vi "ABCD to S - 2nPort.vi"(8 "error in (no error)":errorcluster, 10 "Zc (Ohm)":cdb[](array[numeric]), 11 "ABCD Array In":cdb[][](array[numeric])) -> (0 "error out":errorcluster, 3 "S-par Array Out":cdb[][](array[numeric]))   [LabVIEW 2023, in "NI_HFNetworkAnalysis.lvlib"]
doc: "Convert a 2N-port ABCD array to an S-parameter array, where the characteristic impedance Zc is specified for each port:\n<b>{ b1, b2, b3, b4 } = S . { a1, a2, a3, a4 }</b>\n\nInput ABCD array rows are defined as <b>(a11,a12,a13,a14,...,a21,a22,a23,a24,...,a31,a32,a33,a34,...,a41,a42,a43,a44,...)</b>\nand output S-parameter array rows are defined as <b>(S11,S12,S13,S14,...,S21,S22,S23,S24,...,S31,S32,S33,S34,...,S41,S42,S43,S44,...)</b>.\n\n<b>Note</b>\nThe convention for both S-parameters and ABCD arrays for the current is <b>\"positive when flowing into the port\"</b>.\n\n<b>Known Limitations</b>\nTransformation supports only 2n-port networks."
uses:
  NI_HFNetworkAnalysis.lvlib
  <vilib>/Analysis/baseanly.llb/Complex A x B.vi
  <vilib>/Analysis/Matrix/Numeric/Conversions/Array To Matrix - CA2.vi
  <vilib>/Analysis/baseanly.llb/Complex Inverse Matrix.vi
  <vilib>/Analysis/Matrix/Numeric/Conversions/Matrix To Array - CM.vi
  <vilib>/Analysis/Matrix/NI_Matrix.lvlib
  <vilib>/Analysis/NI_AALBase.lvlib
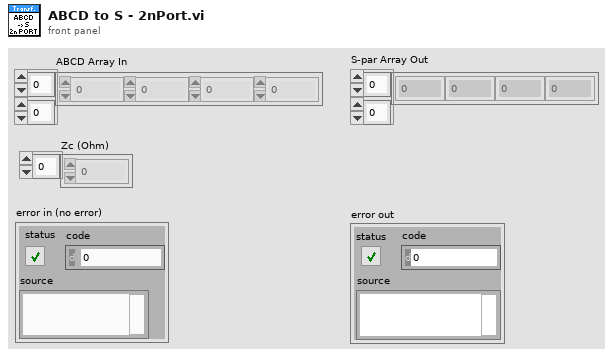
[diagram p1: front panel]
types:
  T1 = typedef "NI_Matrix.lvlib/ComplexMatrix.ctl" = cdb[][]
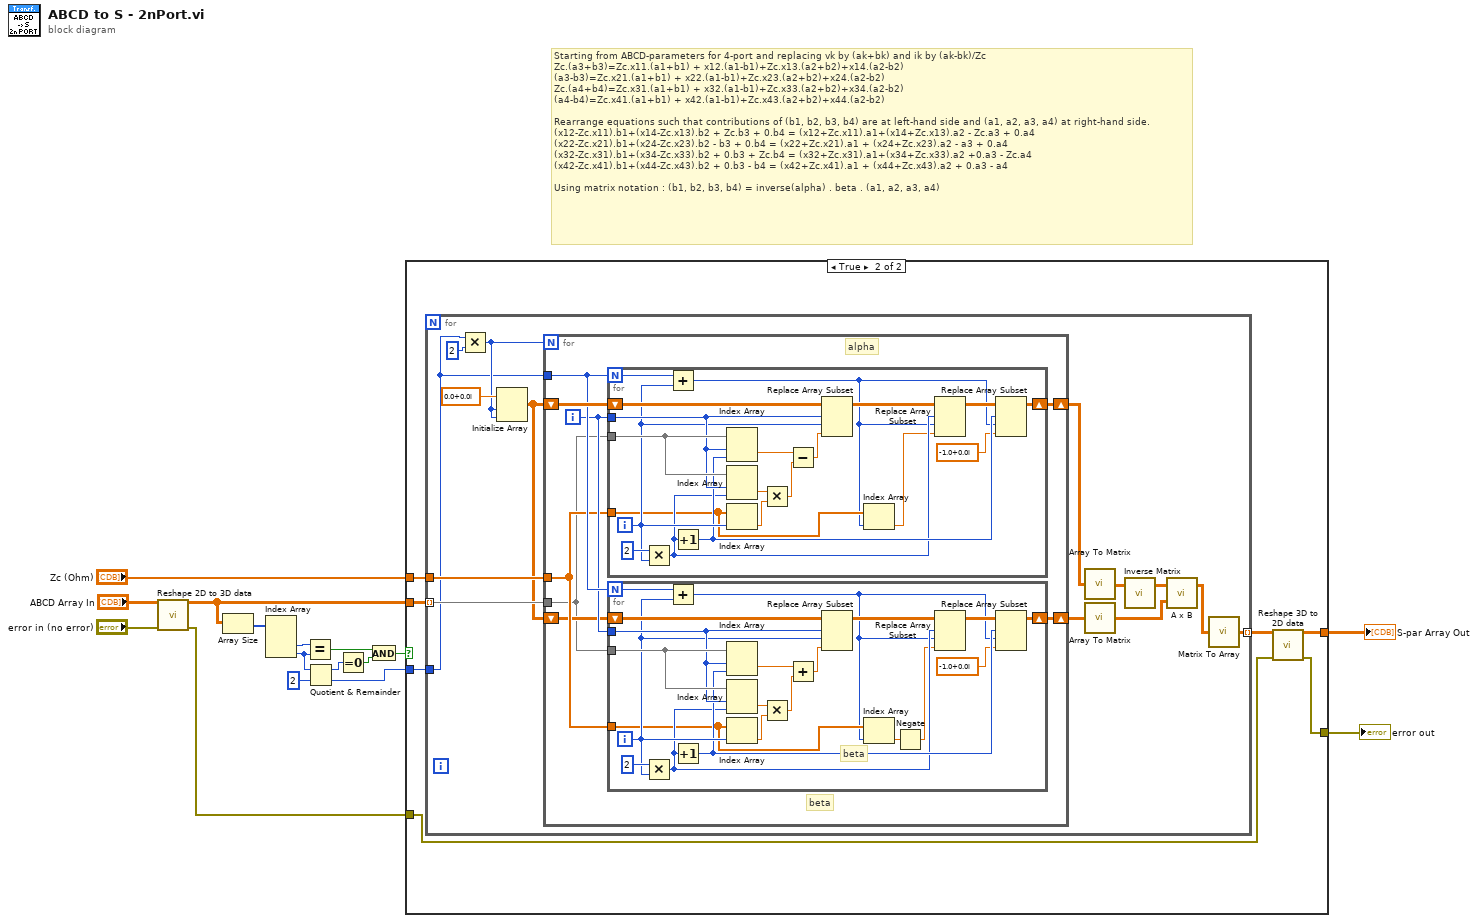
[diagram p0: block diagram]
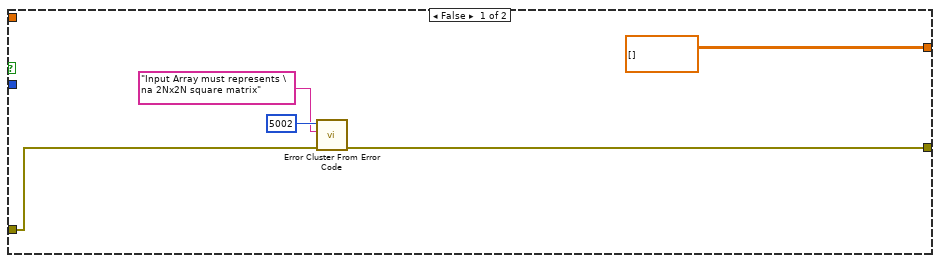
[diagram p2: hidden frame]
diagram:
  # "Starting from ABCD-parameters for 4-port and replacing vk by (ak+bk) and ik by (ak-bk)/Zc\nZc.(a3+b3)=Zc.x11.(a1+b1) + x12.(a1-b1)+Zc.x13.(a2+b2)+x14.(a2-b2)\n(a3-b3)=Zc.x21.(a1+b1) + x22.(a1-b1)+Zc.x23.(a2+b2)+x24.(a2-b2)\nZc.(a4+b4)=Zc.x31.(a1+b1) + x32.(a1-b1)+Zc.x33.(a2+b2)+x34.(a2-b2)\n(a4-b4)=Zc.x41.(a1+b1) + x42.(a1-b1)+Zc.x43.(a2+b2)+x44.(a2-b2)\n\nRearrange equations such that contributions of (b1, b2, b3, b4) are at left-hand side and (a1, a2, a3, a4) at right-hand side.\n(x12-Zc.x11).b1+(x14-Zc.x13).b2 + Zc.b3 + 0.b4 = (x12+Zc.x11).a1+(x14+Zc.x13).a2 - Zc.a3 + 0.a4\n(x22-Zc.x21).b1+(x24-Zc.x23).b2 - b3 + 0.b4 = (x22+Zc.x21).a1 + (x24+Zc.x23).a2 - a3 + 0.a4\n(x32-Zc.x31).b1+(x34-Zc.x33).b2 + 0.b3 + Zc.b4 = (x32+Zc.x31).a1+(x34+Zc.x33).a2 +0.a3 - Zc.a4\n(x42-Zc.x41).b1+(x44-Zc.x43).b2 + 0.b3 - b4 = (x42+Zc.x41).a1 + (x44+Zc.x43).a2 + 0.a3 - a4\n\nUsing matrix notation : (b1, b2, b3, b4) = inverse(alpha) . beta . (a1, a2, a3, a4)"
  n1 = call "Reshape 2D to 3D data.vi"("Parameters In (2D)"="ABCD Array In", "Error In"="error in (no error)") -> ("Parameters Out (3D)"=w15:cdb[][][], "Error Out"=w7:errorcluster)  [unwired: 12 in]
  n2 = Array Size(array=w15) -> (size(s)=w14:i32[])
  n3 = Index Array(array=w14) -> (element #2=w2:i32, element #3=w13:i32)  [unwired: 3 in, 1 out]
  n4 = Equal?(x=w2, y=w13) -> (x = y?=w11:bool)
  n5 = Quotient & Remainder(x=w13, y=2) -> (x-y*floor(x/y)=w4:i32, floor(x/y)=w3:i32)
  n6 = Equal To 0?(x=w4) -> (x = 0?=w10:bool)
  n7 = And(x=w11, y=w10) -> (x .and. y?=w9:bool)
  n8 = case shown="True" w9 {
    tunnel: w15 -> [_ w28]
    tunnel: w3 -> [_ w27]
    tunnel: [cdb[][] [] ("Parameters Out (2D)") w26] -> w8
    tunnel: w7 -> [w20 w23]
    tunnel: [w19 w24] -> w5
    tunnel: "Zc (Ohm)" -> [_ w25]
    frame False {
      n9 = call <vilib>:"Error Cluster From Error Code.vi"("error in (no error)"=w20, "error message (\"\")"="Input Array must represents \na 2Nx2N square matrix" ("error message (\"\")"), "error code (0)"=5002) -> ("error out"=w19:errorcluster)  [unwired: 6 in]
    }
    frame True {
      n10 = for {
        tunnel: w28 -> [w42] mode=indexing
        tunnel: w27 -> [w29]
        tunnel: w25 -> [w39]
        tunnel: [w32] -> w22 mode=indexing
        n11 = Multiply(x=w29, y=2) -> (x*y=w30:i32)
        n12 = Initialize Array(cdb 0.0+0.0i ("element"), w30, w30) -> (w38:cdb[][])
        n13 = for {
          N: w30 -> [_]
          tunnel: w42 -> [w45]
          shift-right: [w43] -> w37
          shift-left: w38 -> [w50]
          tunnel: w29 -> [w49]
          tunnel: w39 -> [w47]
          shift-right: [w44] -> w36
          shift-left: w38 -> [w46]
          i -> [w48]
          # "beta"
          # "beta"
          # "alpha"
          n14 = for {
            N: w49 -> [w79]
            shift-right: [w80] -> w43
            shift-left: w50 -> [w91]
            tunnel: w45 -> [w90]
            tunnel: w48 -> [w89]
            tunnel: w47 -> [w75]
            i -> [w78]
            n15 = Multiply(x=2 ("y"), y=w78) -> (x*y=w76:i32)
            n16 = Add(x=w79, y=w78) -> (x+y=w74:i32)
            n17 = Increment(x=w76) -> (x+1=w77:i32)
            n18 = Index Array(array=w90, index (row)=w89, index (col)=w77) -> (element=w84:cdb)
            n19 = Index Array(array=w90, index (row)=w89, index (col)=w76) -> (element=w86:cdb)
            n20 = Index Array(array=w75, index=w78) -> (element=w87:cdb)
            n21 = Multiply(x=w86, y=w87) -> (x*y=w83:cdb)
            n22 = Subtract(x=w84, y=w83) -> (x-y=w85:cdb)
            n23 = Replace Array Subset(array=w91, new element=w85, index (row)=w89, index (col)=w78) -> (w82:cdb[][])
            n24 = Index Array(array=w75, index=w74) -> (element=w73:cdb)
            n25 = Replace Array Subset(array=w82, new element=w73, index (row)=w76, index (col)=w74) -> (w81:cdb[][])
            n26 = Replace Array Subset(array=w81, new element=cdb -1.0+0.0i ("new element/subarray"), index (row)=w77, index (col)=w74) -> (w80:cdb[][])
          }
          n27 = for {
            N: w49 -> [w59]
            shift-right: [w60] -> w44
            shift-left: w46 -> [w71]
            tunnel: w45 -> [w70]
            tunnel: w48 -> [w69]
            tunnel: w47 -> [w55]
            i -> [w58]
            n28 = Multiply(x=2 ("y"), y=w58) -> (x*y=w56:i32)
            n29 = Add(x=w59, y=w58) -> (x+y=w54:i32)
            n30 = Increment(x=w56) -> (x+1=w57:i32)
            n31 = Index Array(array=w70, index (row)=w69, index (col)=w57) -> (element=w64:cdb)
            n32 = Index Array(array=w70, index (row)=w69, index (col)=w56) -> (element=w66:cdb)
            n33 = Index Array(array=w55, index=w58) -> (element=w67:cdb)
            n34 = Multiply(x=w66, y=w67) -> (x*y=w63:cdb)
            n35 = Add(x=w64, y=w63) -> (x+y=w65:cdb)
            n36 = Replace Array Subset(array=w71, new element=w65, index (row)=w69, index (col)=w58) -> (w62:cdb[][])
            n37 = Index Array(array=w55, index=w54) -> (element=w53:cdb)
            n38 = Negate(x=w53) -> (-x=w51:cdb)
            n39 = Replace Array Subset(array=w62, new element=w51, index (row)=w56, index (col)=w54) -> (w61:cdb[][])
            n40 = Replace Array Subset(array=w61, new element=cdb -1.0+0.0i ("new element/subarray"), index (row)=w57, index (col)=w54) -> (w60:cdb[][])
          }
        }
        n41 = call-poly <vilib>:"Array To Matrix.vi"("Complex 2D Array"=w37) -> ("Complex Matrix"=w35:T1)
        n42 = call-poly <vilib>:"Array To Matrix.vi"("Complex 2D Array"=w36) -> ("Complex Matrix"=w33:T1)
        n43 = call-poly <vilib>:"Inverse Matrix.vi"("Input Matrix"=w35) -> ("Inverse Matrix"=w34:T1)  [unwired: 1 in, 1 out]
        n44 = call-poly <vilib>:"A x B.vi"("B"=w33, "A"=w34) -> ("A x B"=w31:T1)  [unwired: 1 out]
        n45 = call-poly <vilib>:"Matrix To Array.vi"("Complex Matrix"=w31) -> ("Complex 2D Array"=w32:cdb[][])
      }
      n46 = call "Reshape 3D to 2D data.vi"("Parameters In (3D)"=w22, "Error In"=w23) -> ("Parameters Out (2D)"=w26:cdb[][], "Error Out"=w24:errorcluster)  [unwired: 12 in]
    }
  }
  "S-par Array Out" <- w8
  "error out" <- w5
